vi "map_XY_proc_switch.vi"() -> ()   [LabVIEW 2011]
panel:
  in  "Marmo o piastre?":bool
  in  "KILL":bool
  in  "PAUSE":bool
  in  "RESUME":bool
  in  "QUIT":bool
  in  "find z pos 2":bool
  in  "find z pos":bool
  in  "find y pos":bool
  in  "Done":bool
  in  "go to z meas":bool
  in  "find x pos":bool
  in  "zero y":bool
  in  "zero x":bool
  in  "zero Z":bool
  in  "zero done":bool
  out "command":string
  out "output":string
  # "Mappatura a rettangolo\nper marmo e piastre"
  # "ATTENZIONE! \nI valori degli spostamenti  NON\nsono ancora stati aggiornati dopo la\nsostituzione del comparatore!"
  # "In alto: TRUE ---> Marmo"
  # "In basso: FALSE ---> Piastre"
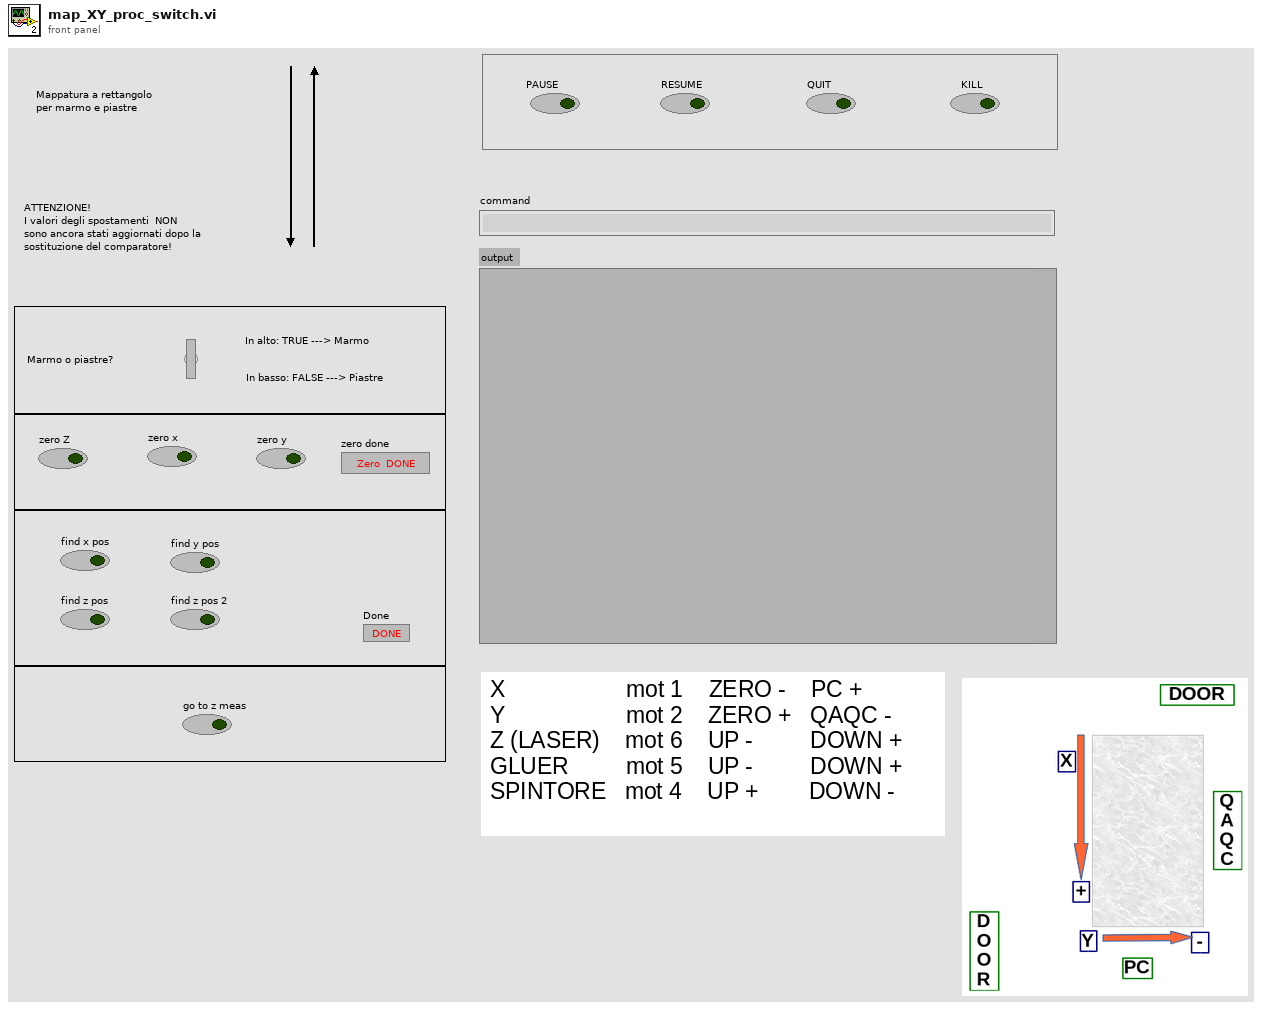
[diagram p1: front panel]
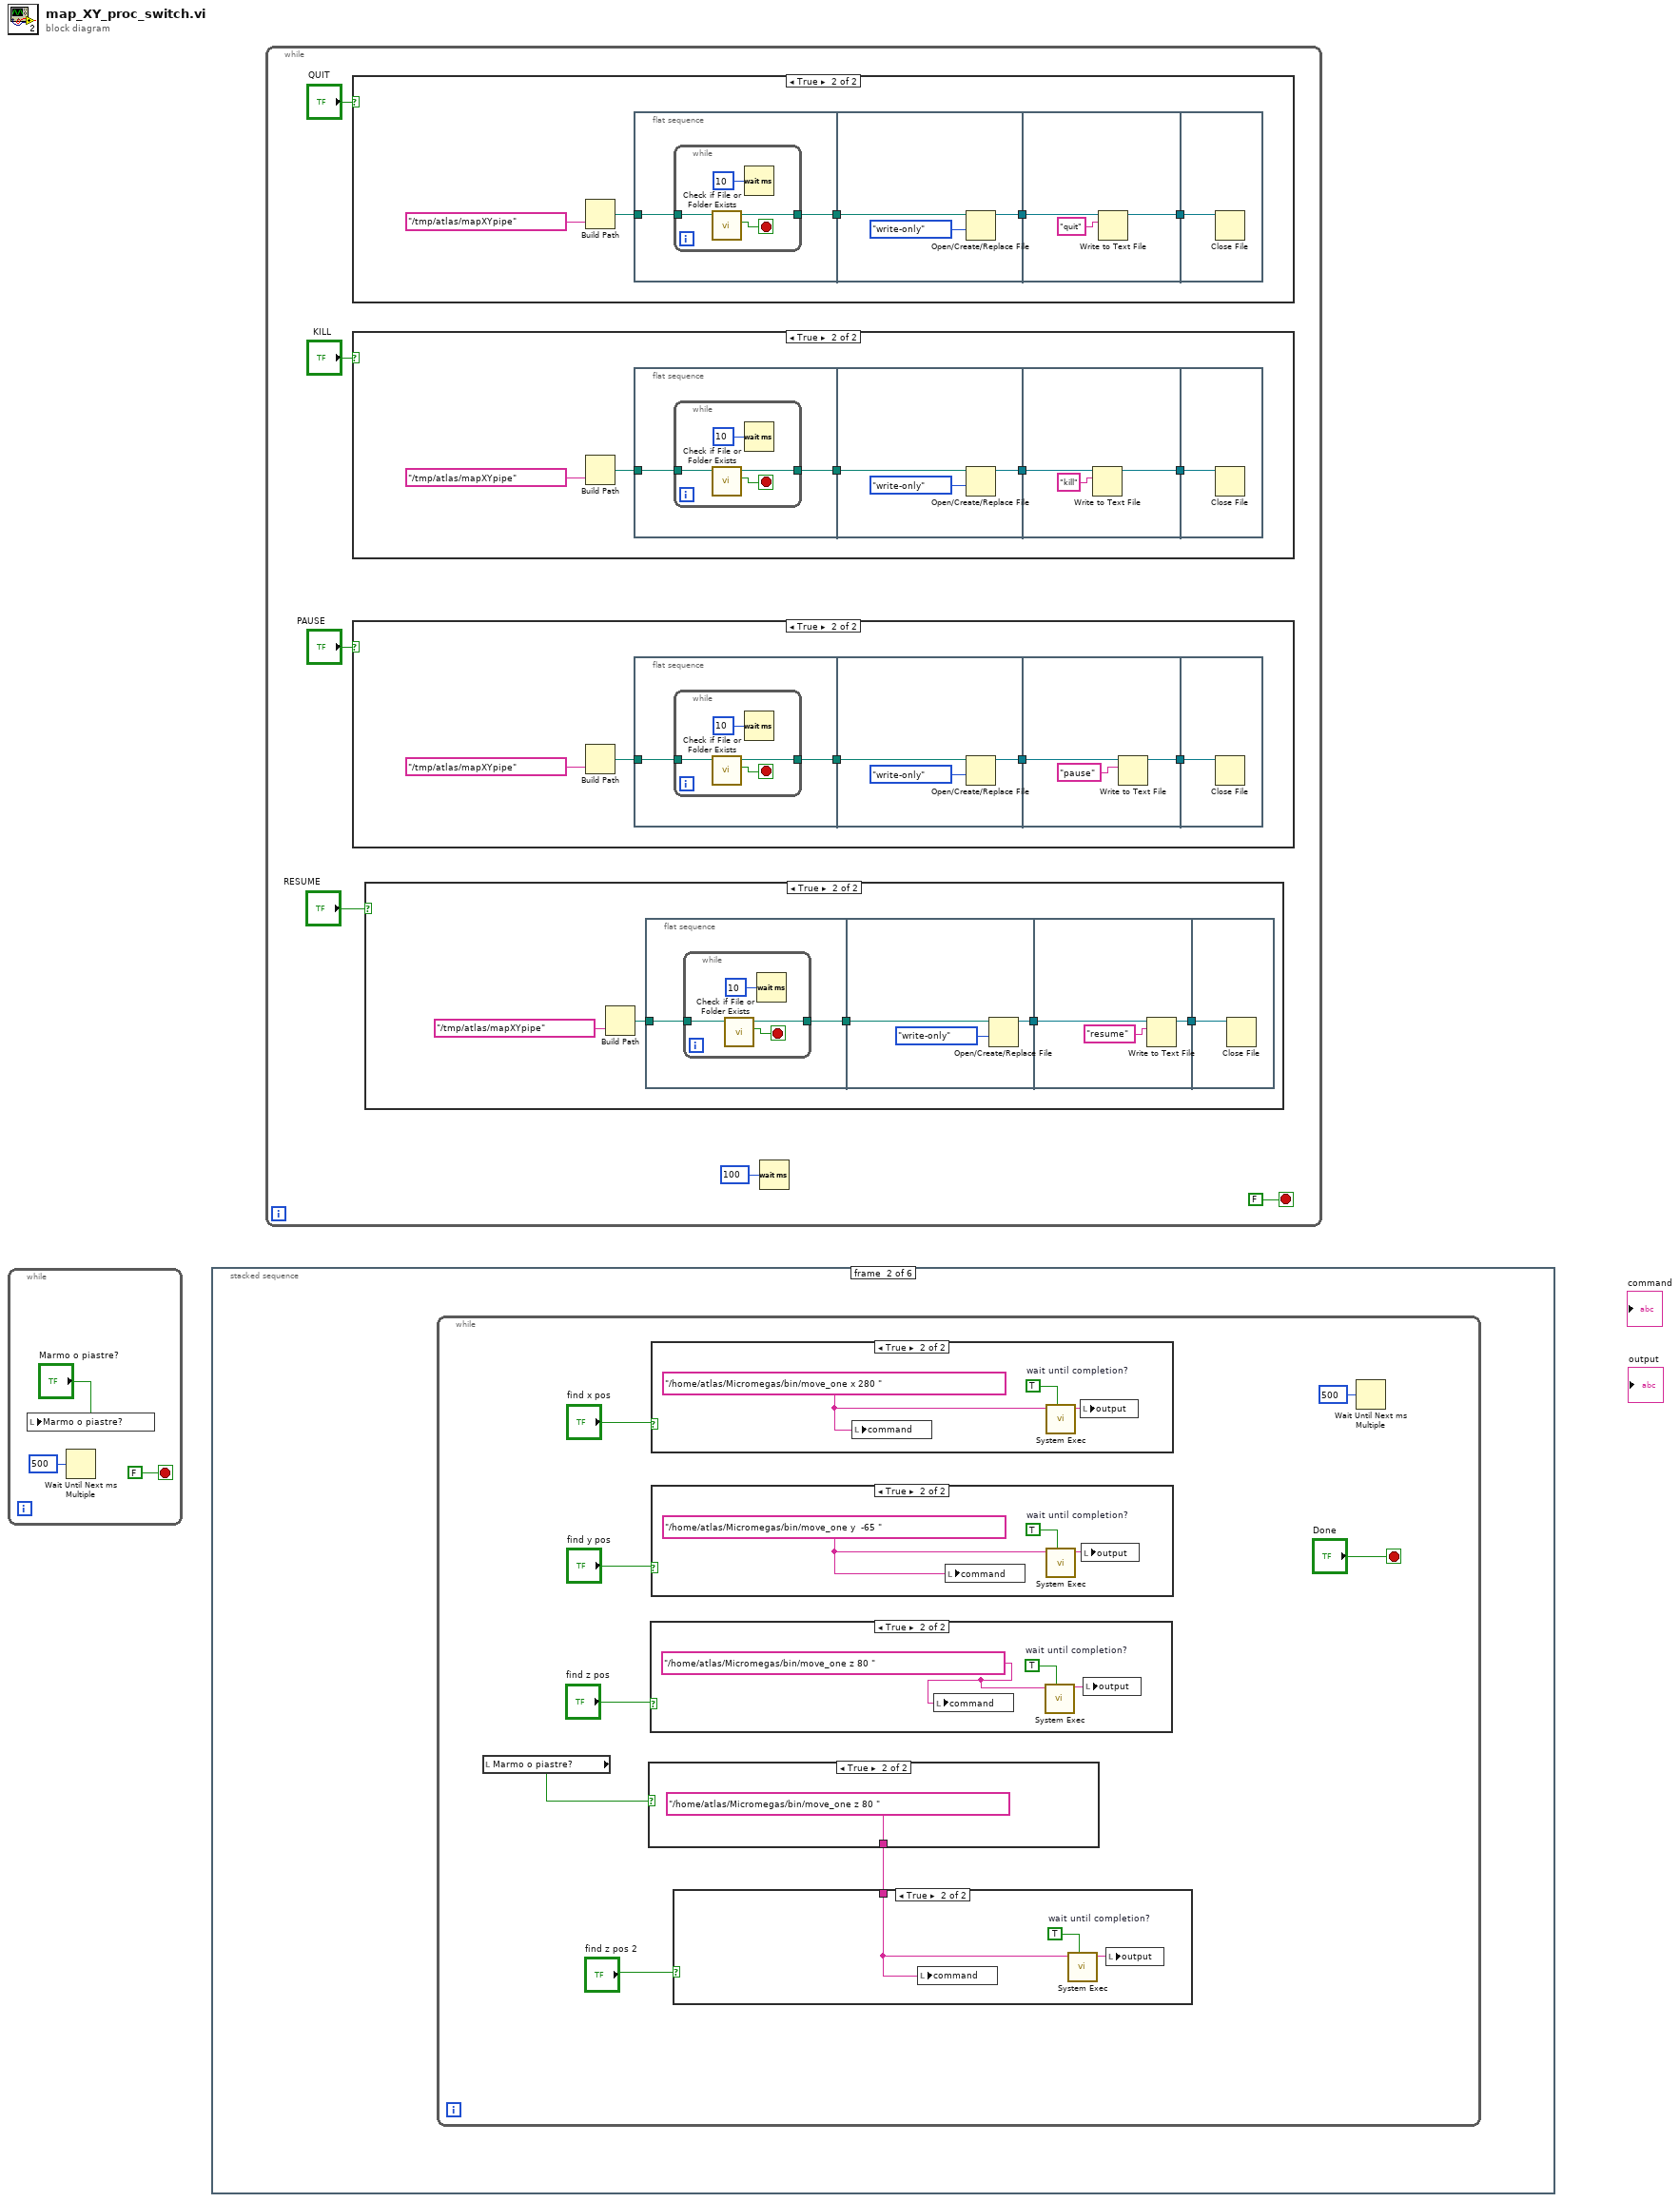
[diagram p0: block diagram]
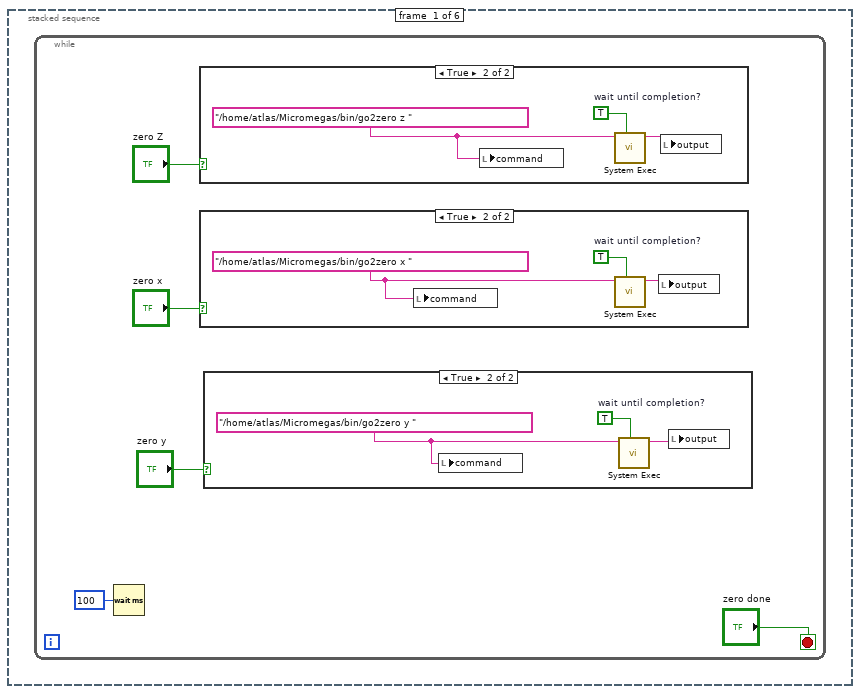
[diagram p6: hidden frame]
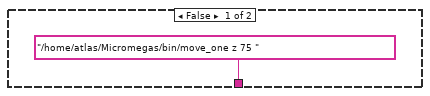
[diagram p10: hidden frame]
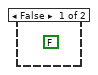
[diagram p12: hidden frame]
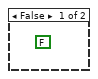
[diagram p13: hidden frame]
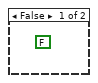
[diagram p14: hidden frame]
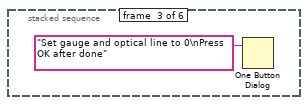
[diagram p15: hidden frame]
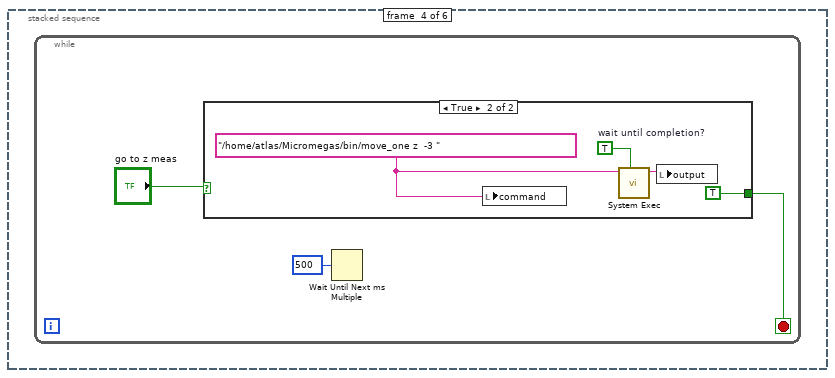
[diagram p16: hidden frame]
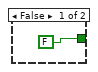
[diagram p17: hidden frame]
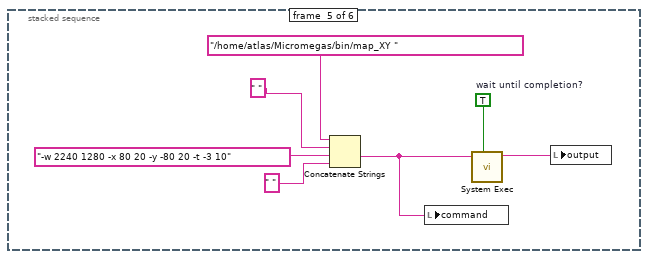
[diagram p18: hidden frame]
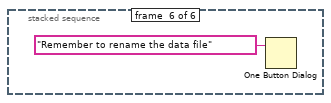
[diagram p19: hidden frame]
diagram:
  n1 = while {
    stop <- FALSE stop-if-true
    n2 = local write "Marmo o piastre?"("Marmo o piastre?") -> ()
    n3 = Wait Until Next ms Multiple(millisecond multiple=u32 500) -> ()  [unwired: 1 out]
  }
  n4 = stacked-sequence {
    frame #0 {
      n5 = while {
        stop <- "zero done" stop-if-true
        n6 = Wait (ms)(milliseconds to wait=u32 100) -> ()  [unwired: 1 out]
        n7 = case shown="True" "zero Z" {
          frame False {
          }
          frame True {
            w16 = "/home/atlas/Micromegas/bin/go2zero z " ("string")
            w17 = TRUE  # wait until completion?
            n8 = local write "command"(w16) -> ()
            n9 = call <vilib>:"System Exec.vi"("wait until completion? (T)"=w17, "command line"=w16) -> ("standard output"=w15:string)  [unwired: 6 in, 3 out]
            n10 = local write "output"(w15) -> ()
          }
        }
        n11 = case shown="True" "zero x" {
          frame False {
          }
          frame True {
            w13 = "/home/atlas/Micromegas/bin/go2zero x " ("string")
            w14 = TRUE  # wait until completion?
            n12 = local write "command"(w13) -> ()
            n13 = call <vilib>:"System Exec.vi"("wait until completion? (T)"=w14, "command line"=w13) -> ("standard output"=w12:string)  [unwired: 6 in, 3 out]
            n14 = local write "output"(w12) -> ()
          }
        }
        n15 = case shown="True" "zero y" {
          frame False {
          }
          frame True {
            w10 = "/home/atlas/Micromegas/bin/go2zero y " ("string")
            w11 = TRUE  # wait until completion?
            n16 = local write "command"(w10) -> ()
            n17 = call <vilib>:"System Exec.vi"("wait until completion? (T)"=w11, "command line"=w10) -> ("standard output"=w9:string)  [unwired: 6 in, 3 out]
            n18 = local write "output"(w9) -> ()
          }
        }
      }
    }
    frame #1 {
      n19 = while {
        stop <- "Done" stop-if-true
        n20 = local read "Marmo o piastre?"() -> (w19:bool)
        n21 = case shown="True" w19 {
          tunnel: ["/home/atlas/Micromegas/bin/move_one z 75 " ("string") "/home/atlas/Micromegas/bin/move_one z 80 " ("string")] -> w20
          frame False {
          }
          frame True {
          }
        }
        n22 = case shown="True" "find z pos" {
          frame False {
            (unwired) FALSE
          }
          frame True {
            w31 = "/home/atlas/Micromegas/bin/move_one z 80 " ("string")
            w33 = TRUE  # wait until completion?
            n23 = local write "command"(w31) -> ()
            n24 = call <vilib>:"System Exec.vi"("wait until completion? (T)"=w33, "command line"=w31) -> ("standard output"=w32:string)  [unwired: 6 in, 3 out]
            n25 = local write "output"(w32) -> ()
          }
        }
        n26 = case shown="True" "find x pos" {
          frame False {
            (unwired) FALSE
          }
          frame True {
            w37 = "/home/atlas/Micromegas/bin/move_one x 280 " ("string")
            w39 = TRUE  # wait until completion?
            n27 = local write "command"(w37) -> ()
            n28 = call <vilib>:"System Exec.vi"("wait until completion? (T)"=w39, "command line"=w37) -> ("standard output"=w38:string)  [unwired: 6 in, 3 out]
            n29 = local write "output"(w38) -> ()
          }
        }
        n30 = case shown="True" "find y pos" {
          frame False {
            (unwired) FALSE
          }
          frame True {
            w34 = "/home/atlas/Micromegas/bin/move_one y  -65 " ("string")
            w36 = TRUE  # wait until completion?
            n31 = local write "command"(w34) -> ()
            n32 = call <vilib>:"System Exec.vi"("wait until completion? (T)"=w36, "command line"=w34) -> ("standard output"=w35:string)  [unwired: 6 in, 3 out]
            n33 = local write "output"(w35) -> ()
          }
        }
        n34 = case shown="True" "find z pos 2" {
          tunnel: w20 -> [_ w28]
          frame False {
          }
          frame True {
            w30 = TRUE  # wait until completion?
            n35 = local write "command"(w28) -> ()
            n36 = call <vilib>:"System Exec.vi"("wait until completion? (T)"=w30, "command line"=w28) -> ("standard output"=w29:string)  [unwired: 6 in, 3 out]
            n37 = local write "output"(w29) -> ()
          }
        }
        n38 = Wait Until Next ms Multiple(millisecond multiple=u32 500) -> ()  [unwired: 1 out]
      }
    }
    frame #2 {
      n39 = One Button Dialog(message="Set gauge and optical line to 0\nPress OK after done") -> ()  [unwired: 1 in, 1 out]
    }
    frame #3 {
      n40 = while {
        stop <- w41 stop-if-true
        n41 = case shown="True" "go to z meas" {
          tunnel: [FALSE TRUE] -> w41
          frame False {
          }
          frame True {
            w47 = "/home/atlas/Micromegas/bin/move_one z  -3 " ("string")
            w48 = TRUE  # wait until completion?
            n42 = local write "command"(w47) -> ()
            n43 = call <vilib>:"System Exec.vi"("wait until completion? (T)"=w48, "command line"=w47) -> ("standard output"=w46:string)  [unwired: 6 in, 3 out]
            n44 = local write "output"(w46) -> ()
          }
        }
        n45 = Wait Until Next ms Multiple(millisecond multiple=u32 500) -> ()  [unwired: 1 out]
      }
    }
    frame #4 {
      w55 = TRUE  # wait until completion?
      n46 = Concatenate Strings("/home/atlas/Micromegas/bin/map_XY " ("string"), " " ("string"), "-w 2240 1280 -x 80 20 -y -80 20 -t -3 10" ("string"), " " ("string")) -> (w53:string)
      n47 = local write "command"(w53) -> ()
      n48 = call <vilib>:"System Exec.vi"("wait until completion? (T)"=w55, "command line"=w53) -> ("standard output"=w52:string)  [unwired: 6 in, 3 out]
      n49 = local write "output"(w52) -> ()
    }
    frame #5 {
      n50 = One Button Dialog(message="Remember to rename the data file") -> ()  [unwired: 1 in, 1 out]
    }
  }
  n51 = while {
    stop <- FALSE stop-if-true
    n52 = case shown="True" "QUIT" {
      frame False {
      }
      frame True {
        n53 = Build Path(name or relative path="/tmp/atlas/mapXYpipe" ("string")) -> (appended path=w117:path)  [unwired: 1 in]
        n54 = flat-sequence {
          tunnel: [w123] -> w121
          tunnel: w117 -> [w122]
          tunnel: w121 -> [w130]
          tunnel: [w128] -> w120
          tunnel: w120 -> [w133]
          tunnel: [w132] -> w119
          tunnel: w119 -> [w134]
          frame #0 {
            n55 = while {
              tunnel: [w125] -> w123
              tunnel: w122 -> [w124]
              stop <- w126 stop-if-true
              n56 = call <vilib>:"Check if File or Folder Exists.vi"("path"=w124) -> ("file or folder exists?"=w126:bool, "dup path"=w125:path)  [unwired: 8 in, 1 out]
              n57 = Wait (ms)(milliseconds to wait=u32 10) -> ()  [unwired: 1 out]
            }
          }
          frame #1 {
            n58 = Open/Create/Replace File(file path (use dialog)=w130, access (0:read/write)=enum16{"read/write", "read-only", "write-only"}."write-only") -> (refnum out=w128:refnum<file>)  [unwired: 4 in, 2 out]
          }
          frame #2 {
            n59 = Write to Text File(file (use dialog)=w133, text="quit") -> (refnum out=w132:refnum<file>)  [unwired: 2 in, 2 out]
          }
          frame #3 {
            n60 = Close File(refnum=w134) -> ()  [unwired: 1 in, 2 out]
          }
        }
      }
    }
    n61 = case shown="True" "KILL" {
      frame False {
      }
      frame True {
        n62 = Build Path(name or relative path="/tmp/atlas/mapXYpipe" ("string")) -> (appended path=w81:path)  [unwired: 1 in]
        n63 = flat-sequence {
          tunnel: [w87] -> w85
          tunnel: w81 -> [w86]
          tunnel: w85 -> [w94]
          tunnel: [w92] -> w84
          tunnel: w84 -> [w97]
          tunnel: [w96] -> w83
          tunnel: w83 -> [w98]
          frame #0 {
            n64 = while {
              tunnel: [w89] -> w87
              tunnel: w86 -> [w88]
              stop <- w90 stop-if-true
              n65 = call <vilib>:"Check if File or Folder Exists.vi"("path"=w88) -> ("file or folder exists?"=w90:bool, "dup path"=w89:path)  [unwired: 8 in, 1 out]
              n66 = Wait (ms)(milliseconds to wait=u32 10) -> ()  [unwired: 1 out]
            }
          }
          frame #1 {
            n67 = Open/Create/Replace File(file path (use dialog)=w94, access (0:read/write)=enum16{"read/write", "read-only", "write-only"}."write-only") -> (refnum out=w92:refnum<file>)  [unwired: 4 in, 2 out]
          }
          frame #2 {
            n68 = Write to Text File(file (use dialog)=w97, text="kill") -> (refnum out=w96:refnum<file>)  [unwired: 2 in, 2 out]
          }
          frame #3 {
            n69 = Close File(refnum=w98) -> ()  [unwired: 1 in, 2 out]
          }
        }
      }
    }
    n70 = case shown="True" "PAUSE" {
      frame False {
      }
      frame True {
        n71 = Build Path(name or relative path="/tmp/atlas/mapXYpipe" ("string")) -> (appended path=w63:path)  [unwired: 1 in]
        n72 = flat-sequence {
          tunnel: [w69] -> w67
          tunnel: w63 -> [w68]
          tunnel: w67 -> [w76]
          tunnel: [w74] -> w66
          tunnel: w66 -> [w79]
          tunnel: [w78] -> w65
          tunnel: w65 -> [w80]
          frame #0 {
            n73 = while {
              tunnel: [w71] -> w69
              tunnel: w68 -> [w70]
              stop <- w72 stop-if-true
              n74 = call <vilib>:"Check if File or Folder Exists.vi"("path"=w70) -> ("file or folder exists?"=w72:bool, "dup path"=w71:path)  [unwired: 8 in, 1 out]
              n75 = Wait (ms)(milliseconds to wait=u32 10) -> ()  [unwired: 1 out]
            }
          }
          frame #1 {
            n76 = Open/Create/Replace File(file path (use dialog)=w76, access (0:read/write)=enum16{"read/write", "read-only", "write-only"}."write-only") -> (refnum out=w74:refnum<file>)  [unwired: 4 in, 2 out]
          }
          frame #2 {
            n77 = Write to Text File(file (use dialog)=w79, text="pause") -> (refnum out=w78:refnum<file>)  [unwired: 2 in, 2 out]
          }
          frame #3 {
            n78 = Close File(refnum=w80) -> ()  [unwired: 1 in, 2 out]
          }
        }
      }
    }
    n79 = case shown="True" "RESUME" {
      frame False {
      }
      frame True {
        n80 = Build Path(name or relative path="/tmp/atlas/mapXYpipe" ("string")) -> (appended path=w99:path)  [unwired: 1 in]
        n81 = flat-sequence {
          tunnel: [w105] -> w103
          tunnel: w99 -> [w104]
          tunnel: w103 -> [w112]
          tunnel: [w110] -> w102
          tunnel: w102 -> [w115]
          tunnel: [w114] -> w101
          tunnel: w101 -> [w116]
          frame #0 {
            n82 = while {
              tunnel: [w107] -> w105
              tunnel: w104 -> [w106]
              stop <- w108 stop-if-true
              n83 = call <vilib>:"Check if File or Folder Exists.vi"("path"=w106) -> ("file or folder exists?"=w108:bool, "dup path"=w107:path)  [unwired: 8 in, 1 out]
              n84 = Wait (ms)(milliseconds to wait=u32 10) -> ()  [unwired: 1 out]
            }
          }
          frame #1 {
            n85 = Open/Create/Replace File(file path (use dialog)=w112, access (0:read/write)=enum16{"read/write", "read-only", "write-only"}."write-only") -> (refnum out=w110:refnum<file>)  [unwired: 4 in, 2 out]
          }
          frame #2 {
            n86 = Write to Text File(file (use dialog)=w115, text="resume") -> (refnum out=w114:refnum<file>)  [unwired: 2 in, 2 out]
          }
          frame #3 {
            n87 = Close File(refnum=w116) -> ()  [unwired: 1 in, 2 out]
          }
        }
      }
    }
    n88 = Wait (ms)(milliseconds to wait=100) -> ()  [unwired: 1 out]
  }
